vi "If statement else end index finder V2.vi"(11 "Auto Scripting array":T1) -> (2 "end Index":i32, 3 "else Index":i32)   [LabVIEW 2013]
uses:
  Autonmous Scripting array typedef.ctl
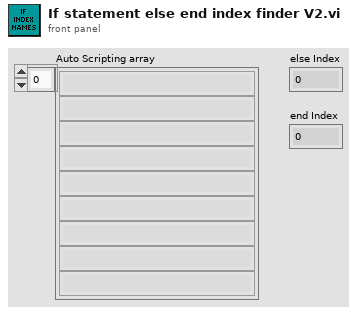
[diagram p1: front panel]
types:
  T1 = typedef "Autonmous Scripting array typedef.ctl" = string[]
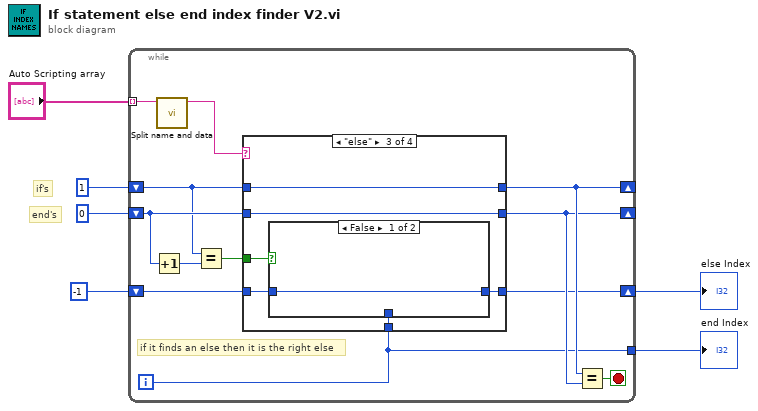
[diagram p0: block diagram]
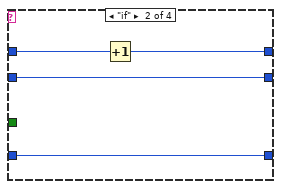
[diagram p3: hidden frame]
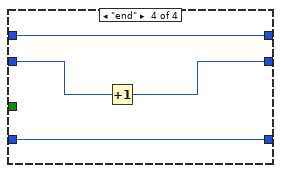
[diagram p5: hidden frame]
diagram:
  # "end's"
  # "if's"
  n1 = while {
    tunnel: "Auto Scripting array" -> [w18] mode=indexing
    shift-right: [w16] -> _
    shift-left: 1 -> [w11]
    shift-right: [w14] -> _
    shift-left: 0 -> [w13]
    tunnel: [w9] -> w4
    shift-right: [w8] -> w5
    shift-left: -1 -> [w7]
    i -> [w9]
    stop <- w15 stop-if-true
    # "if it finds an else then it is the right else"
    n2 = Increment(x=w13) -> (x+1=w12:i32)
    n3 = call "Split name and data.vi"("string"=w18) -> ("Command Name"=w17:string)  [unwired: 9 in, 1 out]
    n4 = Equal?(x=w11, y=w12) -> (x = y?=w10:bool)
    n5 = case shown="\"else\"" w17 {
      tunnel: w11 -> [w21 w24 w31 w37]
      tunnel: w13 -> [w20 w25 w30 w36]
      tunnel: [w21 w23 w31 w37] -> w16
      tunnel: [w20 w25 w30 w35] -> w14
      tunnel: w10 -> [_ _ w29 _]
      tunnel: w9 -> [_ _ w28 _]
      tunnel: [w19 w22 w27 w34] -> w8
      tunnel: w7 -> [w19 w22 w26 w34]
      frame Default {
      }
      frame "if" {
        n6 = Increment(x=w24) -> (x+1=w23:i32)
      }
      frame "else" {
        n7 = case shown="False" w29 {
          tunnel: w28 -> [_ w33]
          tunnel: [w32 w33] -> w27
          tunnel: w26 -> [w32 _]
          frame False {
          }
          frame True {
          }
        }
      }
      frame "end" {
        n8 = Increment(x=w36) -> (x+1=w35:i32)
      }
    }
    n9 = Equal?(x=w16, y=w14) -> (x = y?=w15:bool)
  }
  "else Index" <- w5
  "end Index" <- w4
